vi "set_params.vi"(0 "ESP301viaTCPIP in":refnum<class "ESP301viaTCPIP.lvclass">, 3 "error in (no error)":errorcluster) -> (7 "ESP301viaTCPIP out":refnum<class "ESP301viaTCPIP.lvclass">, 10 "error out":errorcluster)   [LabVIEW 2019, in "ESP301viaTCPIP.lvlib" / "ESP301viaTCPIP.lvclass"]
uses:
  ESP301viaTCPIP.lvclass
panel:
  in  "OK Button":bool
  in  "timeout":i32=1000
  in  "remote port":u16=5002
  in  "TCP IP address":string="10.152.212.240"
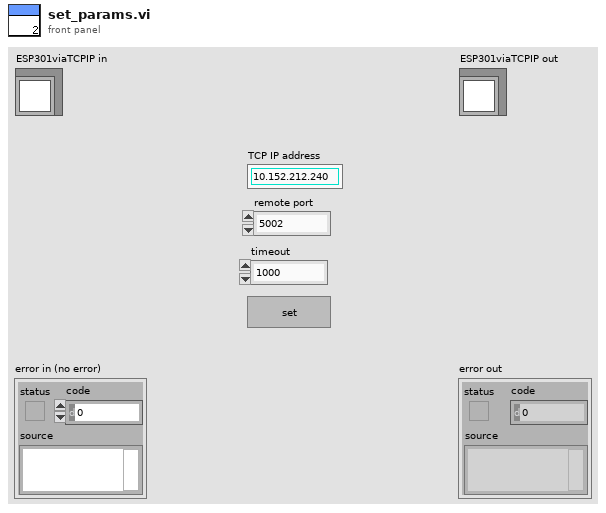
[diagram p1: front panel]
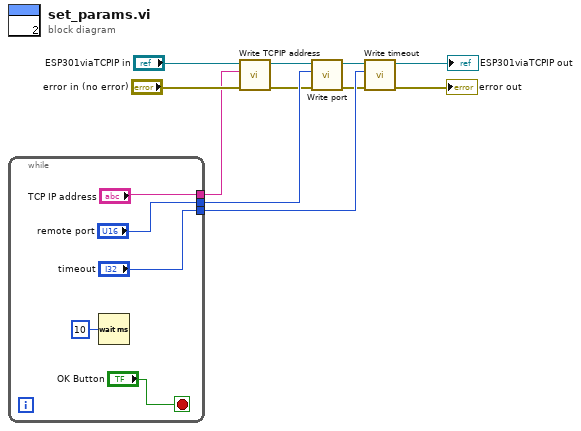
[diagram p0: block diagram]
diagram:
  n1 = while {
    tunnel: ["TCP IP address"] -> w9
    tunnel: ["remote port"] -> w8
    tunnel: ["timeout"] -> w5
    stop <- "OK Button" stop-if-true
    n2 = Wait (ms)(milliseconds to wait=u32 10) -> ()  [unwired: 1 out]
  }
  n3 = call-dynamic "Write TCPIP address.vi"("error in (no error)"="error in (no error)", "TCPIP address"=w9, "ESP301viaTCPIP in"="ESP301viaTCPIP in") -> ("error out"=w6:errorcluster, "ESP301viaTCPIP out"=w7:refnum<class "ESP301viaTCPIP.lvclass">)  [unwired: 7 in]
  n4 = call-dynamic "Write port.vi"("error in (no error)"=w6, "port"=w8, "ESP301viaTCPIP in"=w7) -> ("error out"=w3:errorcluster, "ESP301viaTCPIP out"=w4:refnum<class "ESP301viaTCPIP.lvclass">)  [unwired: 7 in]
  n5 = call-dynamic "Write timeout.vi"("error in (no error)"=w3, "timeout"=w5, "ESP301viaTCPIP in"=w4) -> ("error out"=→"error out":errorcluster, "ESP301viaTCPIP out"=→"ESP301viaTCPIP out":refnum<class "ESP301viaTCPIP.lvclass">)  [unwired: 7 in]
